vi "Tear Down.vi"(8 "error in (no error)":errorcluster, 11 "Bank Account in":refnum<class "Bank Account.lvclass">) -> (0 "error out":errorcluster, 3 "Bank Account out":refnum<class "Bank Account.lvclass">)   [LabVIEW 2016, in "CLD Exam - ATM.lvlib" / "Bank Account.lvclass"]
uses:
  Bank Account.lvclass
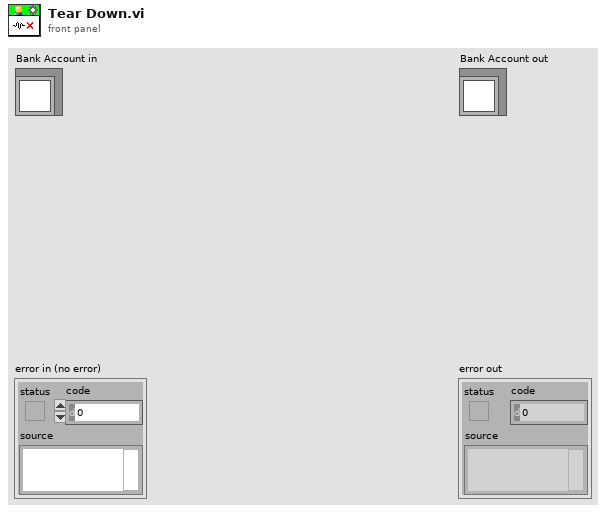
[diagram p1: front panel]
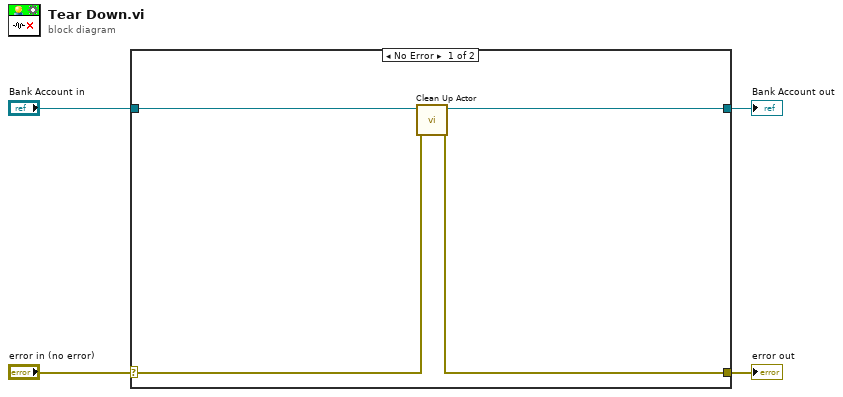
[diagram p0: block diagram]
diagram:
  n1 = case shown="No Error" "error in (no error)" {
    selector: "error in (no error)" -> [w6 w10]
    tunnel: [w5 w10] -> w3
    tunnel: [w7 w9] -> w1
    tunnel: "Bank Account in" -> [w8 w9]
    frame No Error {
      n2 = call-dynamic "Clean Up Actor.vi"("error in (no error)"=w6, "Bank Account in"=w8) -> ("error out"=w5:errorcluster, "Bank Account out"=w7:refnum<class "Bank Account.lvclass">)  [unwired: 8 in]
    }
    frame Error {
    }
  }
  "error out" <- w3
  "Bank Account out" <- w1
